vi "Moyenne_withNaNsuppression.vi"(4 "DBL-Array":sgl[](array[numeric])) -> (0 "Standard Deviation":dbl, 1 "Average":dbl, 2 "Median":dbl)   [LabVIEW 2010]
uses:
  <vilib>/Analysis/NI_AALBase.lvlib
panel:
  out "NaN_index":i32
  out "NaN found?":bool
  out "Exec Time (ms)":u32
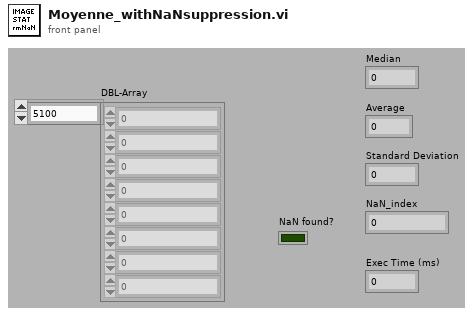
[diagram p1: front panel]
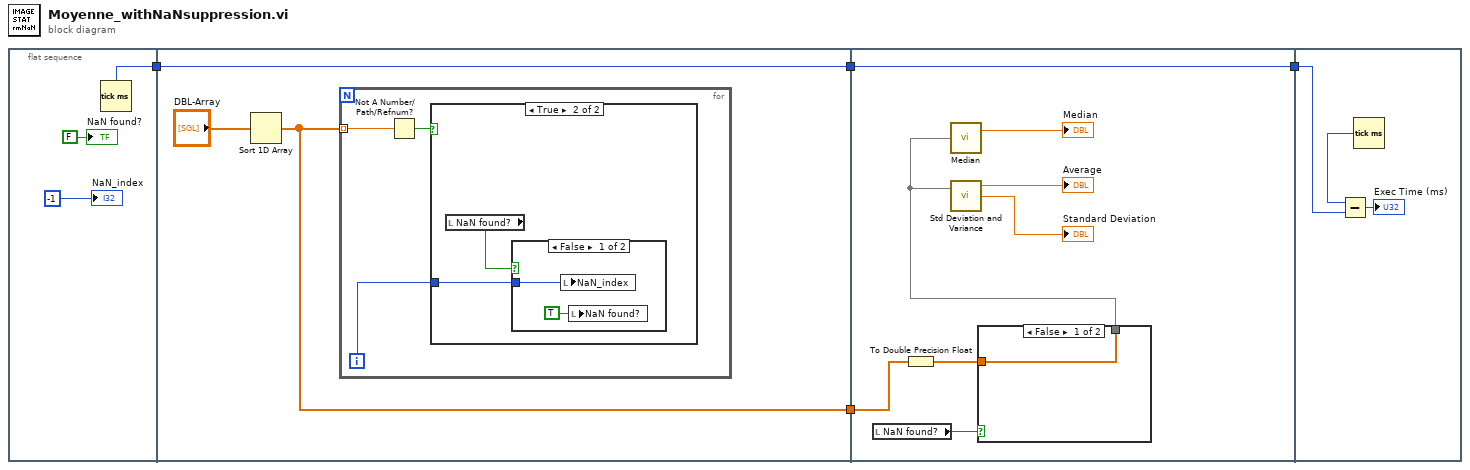
[diagram p0: block diagram]
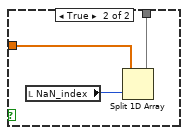
[diagram p4: hidden frame]
diagram:
  n1 = flat-sequence {
    tunnel: [w7] -> w4
    tunnel: w4 -> [w9]
    tunnel: [w9] -> w3
    tunnel: [w8] -> w1
    tunnel: w3 -> [w25]
    tunnel: [w25] -> w2
    tunnel: w1 -> [w23]
    tunnel: w2 -> [w31]
    frame #0 {
      n2 = Tick Count (ms)() -> (millisecond timer value=w7:u32)
      "NaN found?" <- FALSE ("NaN found?")
      "NaN_index" <- -1 ("NaN_index")
    }
    frame #1 {
      n3 = Sort 1D Array(array="DBL-Array") -> (sorted array=w8:sgl[])
      n4 = for {
        tunnel: w8 -> [w12] mode=indexing
        i -> [w11]
        n5 = Not A Number/Path/Refnum?(number/path/refnum=w12) -> (NaN/Path/Refnum?=w13:bool)
        n6 = case shown="True" w13 {
          tunnel: w11 -> [_ w14]
          frame False {
          }
          frame True {
            n7 = local read "NaN found?"() -> (w15:bool)
            n8 = case shown="False" w15 {
              tunnel: w14 -> [w16 _]
              frame False {
                n9 = local write "NaN_index"(w16) -> ()
                n10 = local write "NaN found?"(TRUE ("NaN found?")) -> ()
              }
              frame True {
              }
            }
          }
        }
      }
    }
    frame #2 {
      n11 = local read "NaN found?"() -> (w24:bool)
      n12 = To Double Precision Float(number=w23) -> (double precision float=w18:dbl[])
      n13 = case shown="False" w24 {
        tunnel: w18 -> [w26 w28]
        tunnel: [w26 w27] -> w22
        frame False {
        }
        frame True {
          n14 = local read "NaN_index"() -> (w29:i32)
          n15 = Split 1D Array(array=w28, index=w29) -> (first subarray=w27:dbl[])  [unwired: 1 out]
        }
      }
      n16 = call <vilib>:"Median.vi"("X"=w22) -> ("median"=→"Median":dbl)  [unwired: 1 out]
      n17 = call <vilib>:"Std Deviation and Variance.vi"("X"=w22) -> ("mean"=→"Average":dbl, "standard deviation"=→"Standard Deviation":dbl)  [unwired: 1 in, 1 out]
    }
    frame #3 {
      n18 = Tick Count (ms)() -> (millisecond timer value=w30:u32)
      n19 = Subtract(x=w30, y=w31) -> (x-y=→"Exec Time (ms)":u32)
    }
  }
